vi "Bidirectional Quadrature Decoder .vi"(10 "B":bool, 11 "A":bool) -> (3 "Counter":i32)   [LabVIEW 2018]
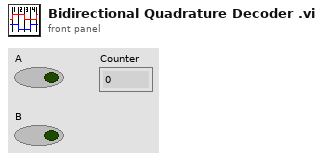
[diagram p1: front panel]
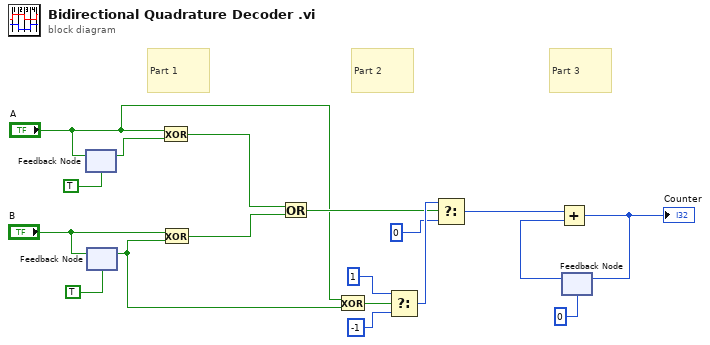
[diagram p0: block diagram]
diagram:
  # "Part 3"
  # "Part 2"
  # "Part 1"
  n1 = feedback #1(TRUE ("A")) -> (w6:bool)
  n2 = feedback-in #1("A") -> ()
  n3 = feedback #2(TRUE ("A")) -> (w4:bool)
  n4 = feedback-in #2("B") -> ()
  n5 = Exclusive Or(1:w6, 2:"A") -> (0:w8:bool)
  n6 = Exclusive Or(1:w4, 2:"B") -> (0:w14:bool)
  n7 = Or(x=w8, y=w14) -> (x .or. y?=w13:bool)
  n8 = Exclusive Or(1:w4, 2:"A") -> (0:w15:bool)
  n9 = Select(t=1, s=w15, f=-1) -> (s? t:f=w18:i32)
  n10 = Select(t=w18, s=w13, f=0) -> (s? t:f=w10:i32)
  n11 = feedback #3(0) -> (w11:i32)
  n12 = Add(x=w10, y=w11) -> (x+y=w12:i32)
  "Counter" <- w12
  n13 = feedback-in #3(w12) -> ()
